vi "Close Client Handle.vi"(8 "error in (no error)":errorcluster, 11 "OAuthClient in":refnum<class "OAuthClient.lvclass">) -> (0 "error out":errorcluster, 3 "OAuthClient out":refnum<class "OAuthClient.lvclass">)   [LabVIEW 2013, in "OAuthClient.lvclass"]
uses:
  OAuthClient.lvclass
  <vilib>/httpClient/ClientHandle.ctl
  OAuthClient.lvclass/OAuthClient.ctl
  <vilib>/httpClient/LabVIEWHTTPClient.lvlib
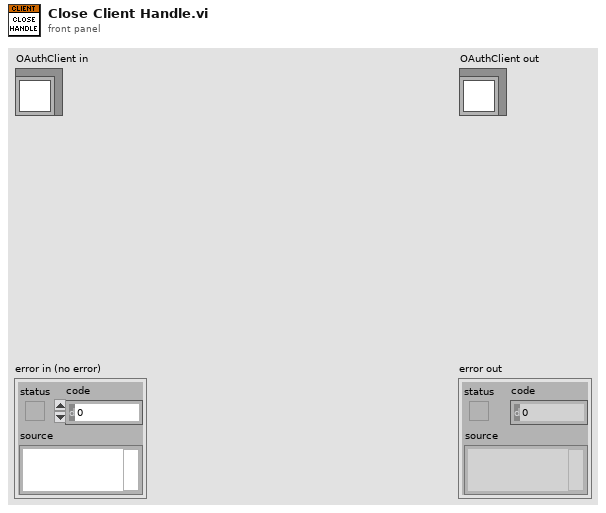
[diagram p1: front panel]
types:
  T1 = typedef "LabVIEWHTTPClient.lvlib/ClientHandle.ctl" = refnum<k1>
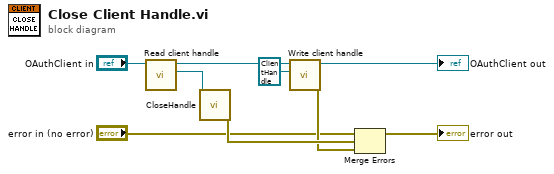
[diagram p0: block diagram]
diagram:
  n1 = call "Read client handle.vi"("OAuthClient in"="OAuthClient in") -> ("Client Handle"=w4:T1, "OAuthClient out"=w5:refnum<class "OAuthClient.lvclass">)  [unwired: 8 in, 1 out]
  n2 = call <vilib>:"CloseHandle.vi"("client handle"=w4) -> ("error out"=w3:errorcluster)  [unwired: 14 in]
  n3 = call "Write client handle.vi"("Client Handle"=T1 refnum, "OAuthClient in"=w5) -> ("error out"=w2:errorcluster, "OAuthClient out"=→"OAuthClient out":refnum<class "OAuthClient.lvclass">)  [unwired: 8 in]
  n4 = Merge Errors("error in (no error)", w3, w2) -> (→"error out":errorcluster)
